vi "Open.vi"(7 "I2C Channel (0)":u8, 8 "Error In":errorcluster, 9 "Resolution":T8, 10 "TCN75A I2C Address":T7, 11 "LINX Resource":T1) -> (0 "Error Out":errorcluster, 3 "LINX Resource":T1)   [LabVIEW 2013, in "LVH-LINX.lvlib" / "TCN75A.lvlib"]
uses:
  <vilib>/LabVIEW Hacker/LINX/Public/Sensors/Temperature/TCN75A/TCN75A.lvlib
  <vilib>/LabVIEW Hacker/LINX/Private/Type Defs/LINX Ref.ctl
  <vilib>/LabVIEW Hacker/LINX/Private/Type Defs/Platform.ctl
  <vilib>/LabVIEW Hacker/LINX/Private/Type Defs/Interface.ctl
  <vilib>/LabVIEW Hacker/LINX/Private/Device/Type Defs/LINX Device Config.ctl
  <vilib>/LabVIEW Hacker/LINX/Private/Device/Type Defs/TCP Config.ctl
  <vilib>/LabVIEW Hacker/LINX/Private/Type Defs/Device Family.ctl
  <vilib>/LabVIEW Hacker/LINX/Public/Sensors/Temperature/TCN75A/Resolution.ctl
  <vilib>/LabVIEW Hacker/LINX/Public/Sensors/Temperature/TCN75A/I2C Address.ctl
  <vilib>/LabVIEW Hacker/LINX/LVH-LINX.lvlib
  <vilib>/LabVIEW Hacker/LINX/Private/Device/Device.lvlib
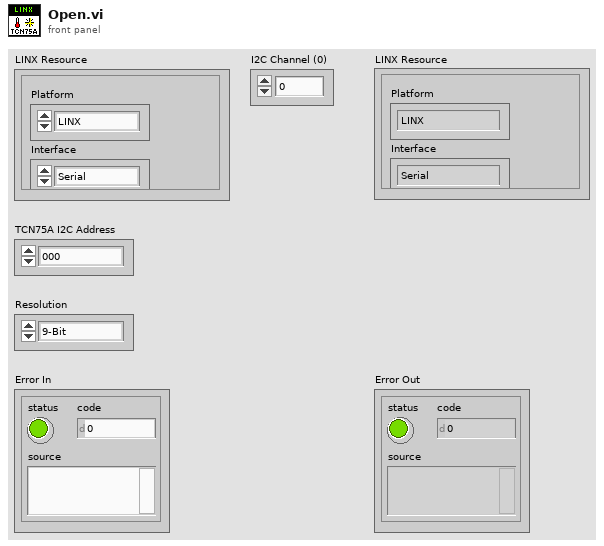
[diagram p1: front panel]
types:
  T1 = typedef "LVH-LINX.lvlib/LINX Ref.ctl" = cluster{"Platform":T2, "Interface":T3, "LINX Device Config":T4}
  T2 = typedef "LVH-LINX.lvlib/Platform.ctl" = enum16{"LINX", "myRIO"}
  T3 = typedef "LVH-LINX.lvlib/Interface.ctl" = enum16{"Serial", "TCP"}
  T4 = typedef "LVH-LINX.lvlib/Device.lvlib/LINX Device Config.ctl" = cluster{"Interface":T3, "COM Port":refnum<visa-resource-name>, "TCP Configuration":T5, "Device Family":T6, "Device ID":u8, "Device Name":string, "TCP Ref":refnum<k5>}
  T5 = typedef "LVH-LINX.lvlib/Device.lvlib/TCP Config.ctl" = cluster{"IP Address":string, "Port":u16}
  T6 = typedef "LVH-LINX.lvlib/Device Family.ctl" = enum8{"National Instruments", "Digilent", "Arduino"}
  T7 = typedef "LVH-LINX.lvlib/TCN75A.lvlib/I2C Address.ctl" = enum8{"000", "001", "010", "011", "100", "101", "110", "111"}
  T8 = typedef "LVH-LINX.lvlib/TCN75A.lvlib/Resolution.ctl" = enum8{"9-Bit", "10-Bit", "11-Bit", "12-Bit"}
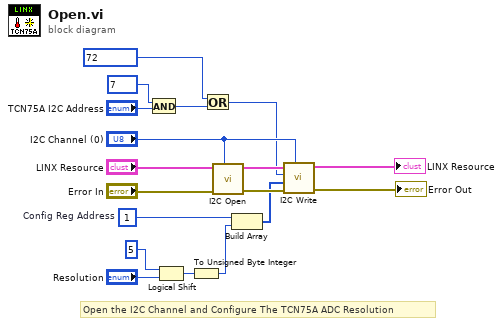
[diagram p0: block diagram]
diagram:
  w5 = u8 1  # Config Reg Address
  # "Open the I2C Channel and Configure The TCN75A ADC Resolution"
  n1 = And(x=u8 7, y="TCN75A I2C Address") -> (x .and. y?=w10:u8)
  n2 = Logical Shift(y=i8 5, x="Resolution") -> (x << y=w14:u32)
  n3 = To Unsigned Byte Integer(number=w14) -> (unsigned 8bit integer=w3:u8)
  n4 = Or(x=u8 72, y=w10) -> (x .or. y?=w6:u8)
  n5 = call <vilib>:"I2C Open.vi"("I2C Channel (0)"="I2C Channel (0)", "Error In"="Error In", "LINX Resource"="LINX Resource") -> ("Error Out"=w8:errorcluster, "LINX Resource"=w9:T1)  [unwired: 7 in]
  n6 = Build Array(w5, w3) -> (w4:u8[])
  n7 = call <vilib>:"I2C Write.vi"("I2C Channel"="I2C Channel (0)", "Error In"=w8, "Data"=w4, "I2C Slave Address (0)"=w6, "LINX Resource"=w9) -> ("Error Out"=→"Error Out":errorcluster, "LINX Resource"=→"LINX Resource":T1)  [unwired: 5 in]
